vi "deleteImpossibleEnemiesToMark.vi"(8 "error in (no error)":errorcluster, 10 "Game":refnum<class "Game.lvclass">, 11 "MarkerSkill in":refnum<class "MarkerSkill.lvclass">) -> (0 "error out":errorcluster, 2 "PossibleEnemiesToMark":refnum<class "Robot.lvclass">[](array[class]), 3 "MarkerSkill out":refnum<class "MarkerSkill.lvclass">)   [LabVIEW 2020, in "MarkerSkill.lvclass"]
uses:
  MarkerSkill.lvclass
  Robot_class/Robot.lvclass
  C:/RoboIME/SSL_AI/Object_class/Object.lvclass
  Game_class/Game.lvclass
  Game_class/Game.lvclass/Game.ctl
  Team_class/Team.lvclass/Team.ctl
  Referee_class/Referee.lvclass/Referee.ctl
  Robot_class/Robot.lvclass/Robot.ctl
  Parameters_class/Parameters.lvclass/Parameters.ctl
  Object_class/Object.lvclass/Object.ctl
  Object_class/Read position(x,y).vi
  Parameters_class/Read DistanceStop.vi
  Game_class/Read EnemyRef.vi
  Game_class/Read Referee.vi
  Game_class/Read BallRef.vi
  Game_class/Read Parameters.lvclass.vi
  Game_class/Read NewParameters.vi
  Game_class/Read OffensiveTeam.vi
  Team_class/Read OffensivePlay.vi
  Referee_class/Read enemy_goalie_id.vi
  Team_class/Read RobotRef.vi
  Robot_class/Read id.vi
  Ally_class/Ally.lvclass
  C:/RoboIME/SSL_AI/Team_class/Team.lvclass
  Enemy_class/Enemy.lvclass
  Ball_class/Ball.lvclass
  Referee_class/Referee.lvclass
  Parameters_class/Parameters.lvclass
  Utilities_class/Utilities.lvclass
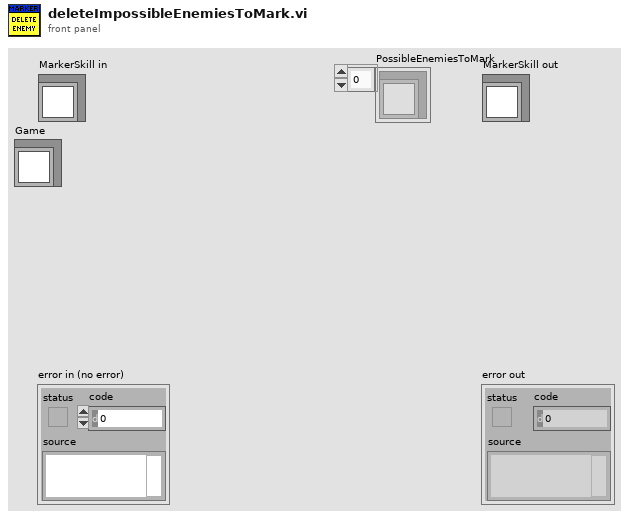
[diagram p1: front panel]
types:
  T1 = typedef "NewParameters.ctl" = cluster{"PenaltyDistance":dbl, "DistanceAttackerToBackBall":dbl, "Division":enum16{"Div B", "Div A"}, "DistanceToAvoidyEnemyRobot":dbl, "BallPlacementDistance":dbl, "DisatanceBehindBallToStealBall":dbl, "MaxDistanceToPositionKickoff":dbl, "BlockEnemyTarget":bool, "MaxStopVAng":dbl, "DistanceMarkerToEnemy":dbl, "IgnoreDribblerContact":bool, "DistanceToBeginEnemyPosession":dbl, "GoToBallWhenEnemyNotMoving":bool, "EnemyDistanceToReduceVelocity":dbl, "TurnOnEnemyDistanceToReduceVelocity":bool, "EnemyDistanceToShootOutBall":dbl, "DefenseKickBall":bool, "MoreKickToGoal? (0-0.3)":dbl, "ChipKickInEnemyField":bool, "ShootOutRobotId":dbl, "FieldLenghtDenominatorInShootOut":dbl, "GoalieKickForce":dbl, "AdjustPositionInBallPlacement":bool, "PowerGodPass":dbl, "VelocityAbortEnemyPos":dbl, "MaxDistToBeginPass":dbl, "MinDistToBeginPass":dbl, "VelocityInDirects":dbl, "BadDribblerIDs":i32[], "NewKickToDistanceAroundBall":dbl, "PowerAvoidColisionMarker":dbl, "DistanceToAvoidColisionMarker":dbl, "AvoidBallKick":dbl, "DistanceTryKick":dbl, "SuicideKickDIstance":dbl, "SuicideKickAtck":bool, "SuicideAngleDistance":dbl, "SuicideKickDefense":bool, "AvoidAimLessKick":dbl, "KIckForceWithChipKick":dbl, "DistanceToAvoidyEnemyShootRobot ":dbl, "NumberOfMarkers":dbl}
  T2 = typedef "OffensivePlay.ctl" = enum16{"5RobotsPassGamePlay", "5PreparePassGame", "5RobotsKeeperGame", "KeeperPassToStriker", "5RobotsNormalGamePlay", "PrepareKeeperPass", "ACBPass", "ABCPass", "PrepareTriplePass", "TableWithStriker", "TableWith2ndStrikerPlay", "PrepareDoublePass", "PrepareRollToPass", "SimplePass", "PreparePass", "PassToStriker", "BallOutOfField", "PassTo2ndStriker", "StopOffensive", "Prepare Penalty Enemy", "EnemyPossessionAtEnemyField", "EnemyPossesionAtOurField", "TestPlay", "PreparePenaltyAlly", "KickPenaltyAlly", "PrepareKickoffAlly", "PrepareKickoffEnemy", "IndirectEnemy", "DirectEnemy", "PreparePassInGame1", "NormalGame", "DirectKick", "Pass", "Halt", "Timeout", "PassPlay", "PenaltyEnemy"}
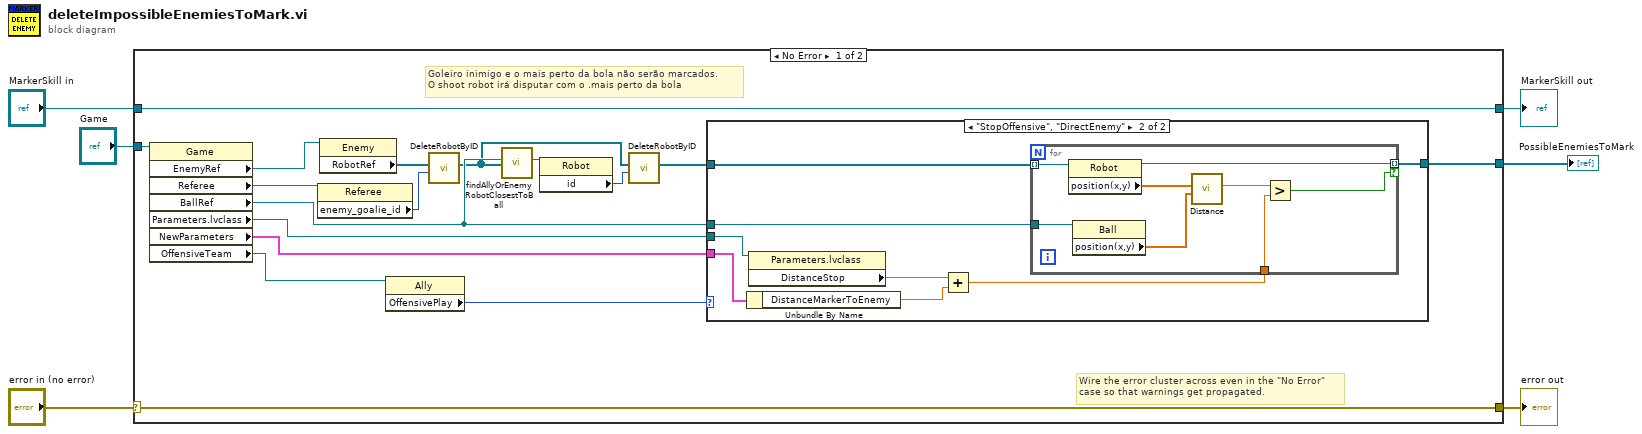
[diagram p0: block diagram]
diagram:
  n1 = case shown="No Error" "error in (no error)" {
    selector: "error in (no error)" -> [w22 w42]
    tunnel: [w22 w42] -> w5
    tunnel: [w23 w41] -> w3
    tunnel: "MarkerSkill in" -> [w23 w41]
    tunnel: [w21 _] -> w2
    tunnel: "Game" -> [w20 _]
    frame No Error {
      # "Goleiro inimigo e o mais perto da bola não serão marcados.\nO shoot robot irá disputar com o .mais perto da bola"
      # "Wire the error cluster across even in the \"No Error\"\ncase so that warnings get propagated."
      n2 = property class="Game"(reference=w20) -> ("EnemyRef"=w19:refnum<class "Enemy.lvclass">, "Referee"=w17:refnum<class "Referee.lvclass">, "BallRef"=w11:refnum<class "Ball.lvclass">, "Parameters.lvclass"=w13:refnum<class "Parameters.lvclass">, "NewParameters"=w14:T1, "OffensiveTeam"=w12:refnum<class "Ally.lvclass">)  [unwired: 1 in, 2 out]
      n3 = property class="Referee"(reference=w17) -> ("enemy_goalie_id"=w16:i32)  [unwired: 1 in, 2 out]
      n4 = property class="Enemy"(reference=w19) -> ("RobotRef"=w18:refnum<class "Robot.lvclass">[])  [unwired: 1 in, 2 out]
      n5 = property class="Ally"(reference=w12) -> ("OffensivePlay"=w15:T2)  [unwired: 1 in, 2 out]
      n6 = call "DeleteRobotByID.vi"("id"=w16, "RobotRef"=w18) -> ("RobotRef out"=w8:refnum<class "Robot.lvclass">[])  [unwired: 7 in, 2 out]
      n7 = call "findAllyOrEnemyRobotClosestToBall.vi"("Ally/Enemy Robots"=w8, "Ball"=w11) -> ("Robot"=w10:refnum<class "Robot.lvclass">)  [unwired: 6 in, 3 out]
      n8 = property class="Robot"(reference=w10) -> ("id"=w9:i32)  [unwired: 1 in, 2 out]
      n9 = call "DeleteRobotByID.vi"("id"=w9, "RobotRef"=w8) -> ("RobotRef out"=w7:refnum<class "Robot.lvclass">[])  [unwired: 7 in, 2 out]
      n10 = case shown="\"StopOffensive\", \"DirectEnemy\"" w15 {
        tunnel: w7 -> [w24 w32]
        tunnel: [w24 w31] -> w21
        tunnel: w11 -> [_ w30]
        tunnel: w14 -> [_ w27]
        tunnel: w13 -> [_ w26]
        frame Default {
        }
        frame "StopOffensive", "DirectEnemy" {
          n11 = Unbundle By Name(w27) -> ("DistanceMarkerToEnemy"=w29:dbl)
          n12 = property class="Parameters.lvclass"(reference=w26) -> ("DistanceStop"=w28:dbl)  [unwired: 1 in, 2 out]
          n13 = Add(x=w28, y=w29) -> (x+y=w25:dbl)
          n14 = for {
            tunnel: w32 -> [w40] mode=indexing
            tunnel: [w39] -> w31 mode=indexing if=w35
            tunnel: w30 -> [w34]
            tunnel: w25 -> [w33]
            n15 = property class="Robot"(reference=w40) -> (reference out=w39:refnum<class "Robot.lvclass">, "position(x,y)"=w38:dbl[])  [unwired: 1 in, 1 out]
            n16 = property class="Ball"(reference=w34) -> ("position(x,y)"=w37:dbl[])  [unwired: 1 in, 2 out]
            n17 = call "Distance.vi"("P1"=w37, "P2"=w38) -> ("Distance"=w36:dbl)  [unwired: 7 in, 2 out]
            n18 = Greater?(x=w36, y=w33) -> (0:w35:bool)
          }
        }
      }
    }
    frame Error {
    }
  }
  "error out" <- w5
  "MarkerSkill out" <- w3
  "PossibleEnemiesToMark" <- w2
